vi "LWXPS_Example_ZygoAmplitudeGet.vi"() -> ()   [LabVIEW 2013]
panel:
  out "Error out":errorcluster caption="error out"
  out "Measuring channel amplitude 2":i32
  out "Measuring channel amplitude 1":i32
  out "Zygo reference signal status":i32
  in  "Instrument Key IN":string
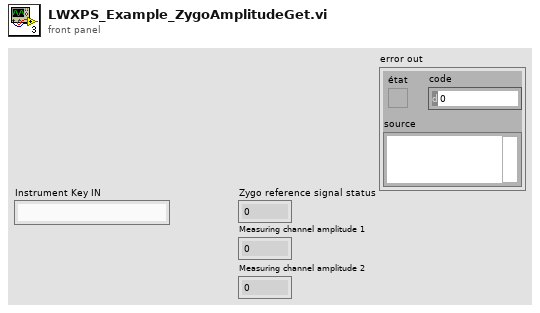
[diagram p1: front panel]
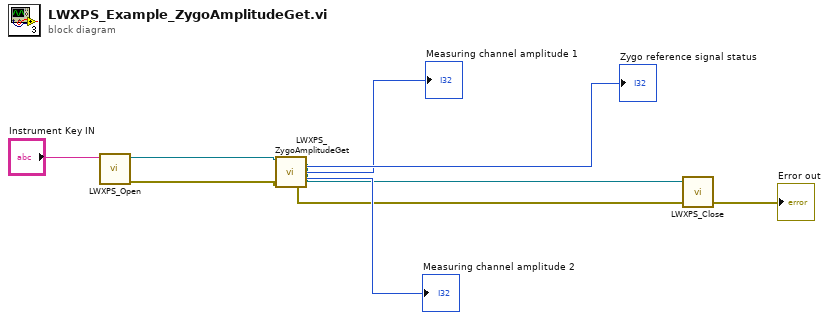
[diagram p0: block diagram]
diagram:
  n1 = call "LWXPS_Open.vi"("Instrument Key IN"="Instrument Key IN") -> ("error out"=w7:errorcluster, "CommandInterfaceXPS.XPS"=w8:refnum<k24>)  [unwired: 3 in, 2 out]
  n2 = call "LWXPS_ZygoAmplitudeGet.vi"("XPS Reference IN"=w8, "LabVIEW error IN"=w7) -> ("CommandInterfaceXPS.XPS"=w3:refnum<k24>, "Zygo reference signal status"=→"Zygo reference signal status":i32, "Measuring channel amplitude 1"=→"Measuring channel amplitude 1":i32, "Measuring channel amplitude 2"=→"Measuring channel amplitude 2":i32, "LabVIEW error OUT"=w2:errorcluster)  [unwired: 7 in, 2 out]
  n3 = call "LWXPS_Close.vi"("error in (no error)"=w2, "XPS Reference"=w3) -> ("Error out"=→"Error out":errorcluster)  [unwired: 2 in, 1 out]
